vi "record_AnMiTC_to_tsv.vi"(7 "folder_name":string="Anneal_Microwave_TC", 9 "temperatures":dbl[](array[numeric])=[0.0], 10 "time":timestamp, 11 "file_name":string="record") -> ()   [LabVIEW 2019]
uses:
  <vilib>/Utility/file.llb/Write Delimited Spreadsheet (string).vi
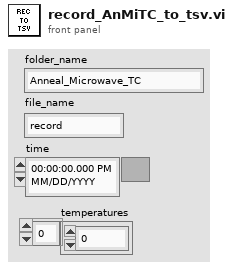
[diagram p1: front panel]
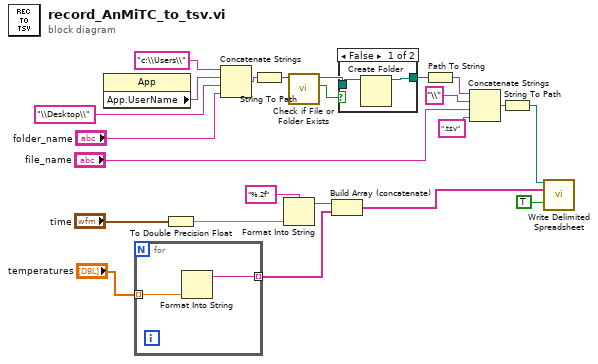
[diagram p0: block diagram]
diagram:
  n1 = property class="App"() -> ("App.UserName"=w19:string)  [unwired: 2 in, 2 out]
  n2 = for {
    tunnel: [w25] -> w1 mode=indexing
    tunnel: "temperatures" -> [w24] mode=indexing
    n3 = Format Into String(w24) -> (resulting string=w25:string)  [unwired: 3 in, 1 out]
  }
  n4 = To Double Precision Float(number="time") -> (double precision float=w4:dbl)
  n5 = Concatenate Strings("c:\\Users\\", w19, "\\Desktop\\", "folder_name") -> (w17:string)
  n6 = String To Path(string=w17) -> (path=w12:path)
  n7 = Format Into String(format string="%.2f", w4) -> (resulting string=w23:string)  [unwired: 2 in, 1 out]
  n8 = call <vilib>:"Check if File or Folder Exists.vi"("path"=w12) -> ("file or folder exists?"=w11:bool, "dup path"=w9:path)  [unwired: 8 in, 1 out]
  n9 = Build Array (concatenate)(w23, w1) -> (w22:string[])
  n10 = case shown="False" w11 {
    tunnel: w9 -> [w27 w28]
    tunnel: [w26 w28] -> w10
    frame False {
      n11 = Create Folder(path (use dialog)=w27) -> (created path=w26:path)  [unwired: 2 in, 2 out]
    }
    frame True {
    }
  }
  n12 = Path To String(path=w10) -> (string=w8:string)
  n13 = Concatenate Strings(w8, "\\", "file_name", ".tsv" ("string")) -> (w13:string)
  n14 = String To Path(string=w13) -> (path=w7:path)
  n15 = call-poly <vilib>:"Write Delimited Spreadsheet.vi"("file path (dialog if empty)"=w7, "1D data"=w22, "append to file? (new file:F)"=TRUE) -> ()  [unwired: 11 in, 2 out]
